vi "writeStatesSamples.vi"(0 "Game in":refnum<class "Game.lvclass">, 1 "Start Recording":bool, 2 "Clear":bool, 3 "Dump":bool, 5 "error in (no error)":errorcluster, 6 "RobotModelFolder":string, 8 "uk":dbl[](array[numeric])) -> (14 "Game out":refnum<class "Game.lvclass">, 19 "error out":errorcluster)   [LabVIEW 2020, in "Game.lvclass"]
uses:
  Game.lvclass
  Game.lvclass/Game.ctl
  Team_class/Team.lvclass/Team.ctl
  Object_class/Object.lvclass/Object.ctl
  Robot_class/Robot.lvclass/Robot.ctl
  Read AllyRef.vi
  Team_class/Read RobotRef.vi
  Object_class/Read x.vi
  Object_class/Read y.vi
  Robot_class/Read orientation.vi
  Ally_class/Ally.lvclass
  C:/Users/anton/Desktop/RoboIME/IC/SSL_AI/Team_class/Team.lvclass
  Robot_class/Robot.lvclass
  C:/Users/anton/Desktop/RoboIME/IC/SSL_AI/Object_class/Object.lvclass
  Utilities_class/Utilities.lvclass
panel:
  out "output array":dbl[][](array[numeric])
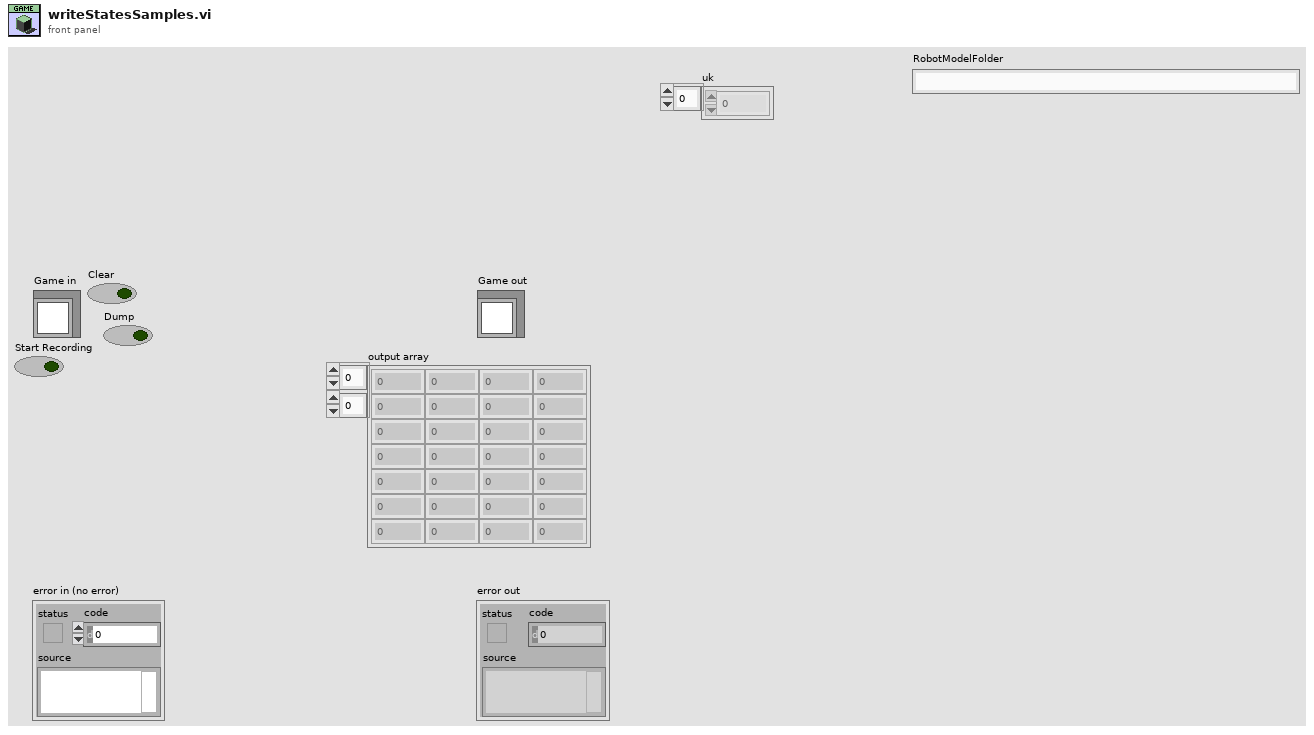
[diagram p1: front panel]
types:
  T1 = cluster{"signal":dbl, "signal":dbl, "signal":dbl}
  T2 = cluster{"signal":dbl, "signal":dbl, "signal":dbl}[]
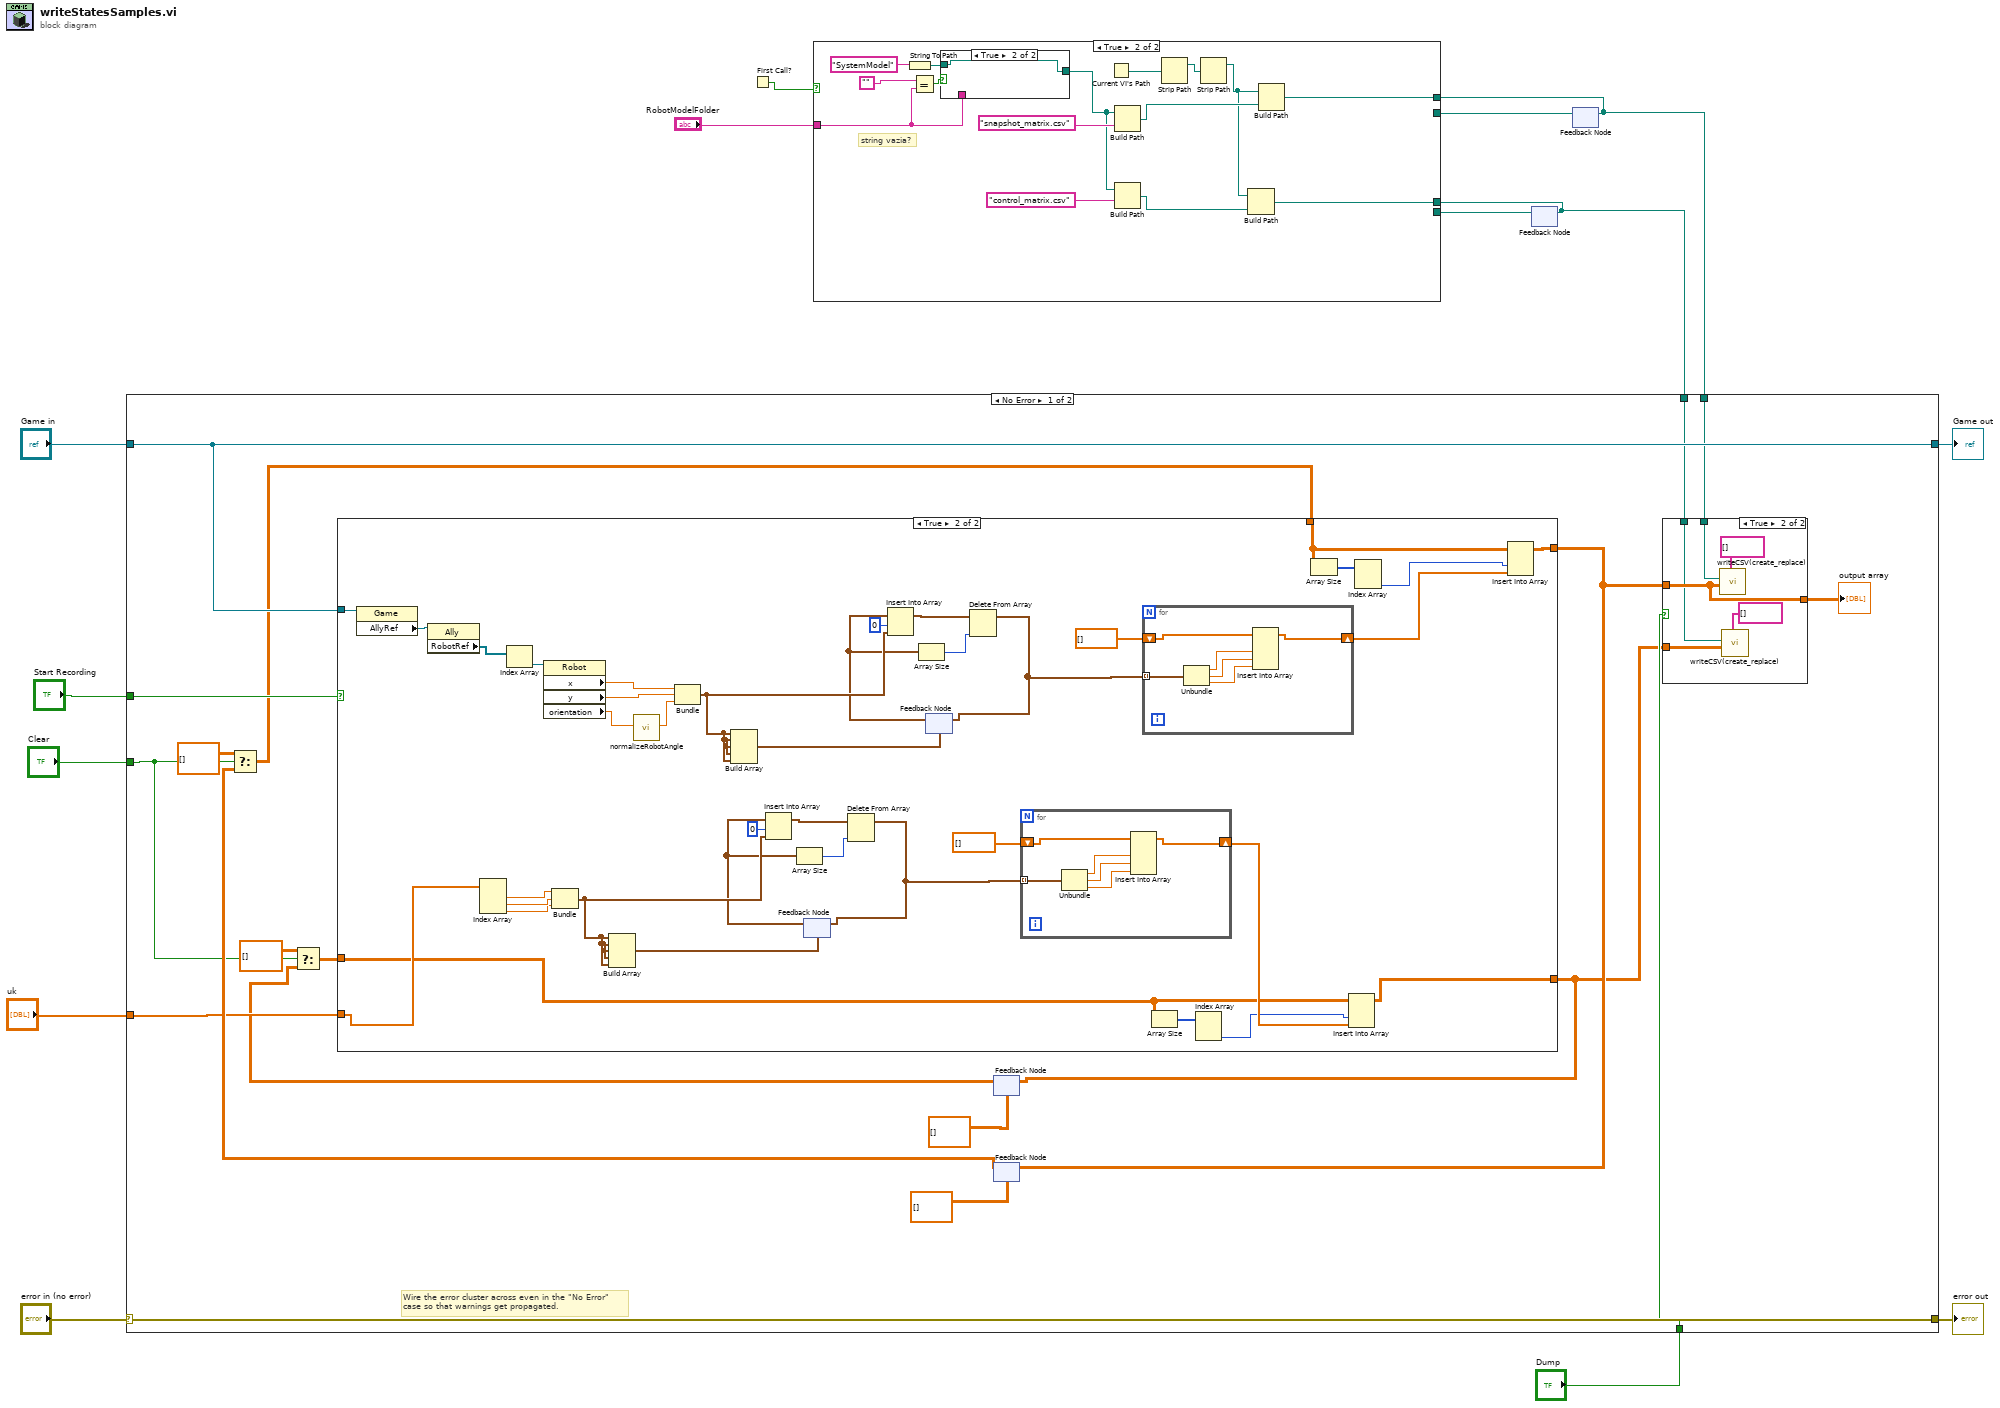
[diagram p0: block diagram]
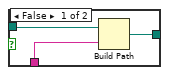
[diagram p3: hidden frame]
diagram:
  n1 = First Call?() -> (First Call?: T/F=w8:bool)
  n2 = feedback #1() -> (w2:path)  [unwired: 1 in]
  n3 = feedback #2() -> (w6:path)  [unwired: 1 in]
  n4 = case shown="True" w8 {
    tunnel: [w16 w29] -> w4
    tunnel: "RobotModelFolder" -> [_ w22]
    tunnel: w6 -> [w16 _]
    tunnel: [w15 w17] -> w1
    tunnel: w2 -> [w15 _]
    frame False {
      # "só precisa calcular o path na 1° iteração"
    }
    frame True {
      # "string vazia?"
      n5 = String To Path(string="SystemModel" ("name or relative path")) -> (path=w23:path)
      n6 = Equal?(x="", y=w22) -> (x = y?=w26:bool)
      n7 = case shown="True" w26 {
        tunnel: w22 -> [w34 _]
        tunnel: [w33 w35] -> w21
        tunnel: w23 -> [w32 w35]
        frame False {
          n8 = Build Path(base path=w32, name or relative path=w34) -> (appended path=w33:path)
        }
        frame True {
        }
      }
      n9 = Current VI's Path() -> (path=w31:path)
      n10 = Build Path(base path=w21, name or relative path="snapshot_matrix.csv") -> (appended path=w27:path)
      n11 = Build Path(base path=w21, name or relative path="control_matrix.csv") -> (appended path=w19:path)
      n12 = Strip Path(path=w31) -> (stripped path=w30:path)  [unwired: 1 out]
      n13 = Strip Path(path=w30) -> (stripped path=w18:path)  [unwired: 1 out]
      n14 = Build Path(base path=w18, name or relative path=w19) -> (appended path=w17:path)
      n15 = Build Path(base path=w18, name or relative path=w27) -> (appended path=w29:path)
    }
  }
  n16 = case shown="No Error" "error in (no error)" {
    selector: "error in (no error)" -> [w54 w115]
    tunnel: [w54 w115] -> w13
    tunnel: [w53 w114] -> w11
    tunnel: "Game in" -> [w53 w114]
    tunnel: "Start Recording" -> [w51 _]
    tunnel: "Clear" -> [w41 _]
    tunnel: "Dump" -> [w48 _]
    tunnel: w4 -> [w47 _]
    tunnel: "uk" -> [w43 _]
    tunnel: w1 -> [w37 _]
    frame No Error {
      # "Wire the error cluster across even in the \"No Error\"\ncase so that warnings get propagated."
      n17 = feedback #3(dbl[][] [] ("appended array")) -> (w40:dbl[][])
      n18 = Select(t=dbl[][] [], s=w41, f=w40) -> (s? t:f=w38:dbl[][])
      n19 = feedback #4(dbl[][] [] ("appended array")) -> (w44:dbl[][])
      n20 = Select(t=dbl[][] [], s=w41, f=w44) -> (s? t:f=w49:dbl[][])
      n21 = case shown="True" w51 {
        tunnel: w53 -> [_ w101]
        tunnel: [w63 w87] -> w46
        tunnel: w49 -> [w63 w86]
        tunnel: w43 -> [_ w69]
        tunnel: w38 -> [w62 w65]
        tunnel: [w62 w64] -> w36
        frame False {
        }
        frame True {
          n22 = property class="Game"(reference=w101) -> ("AllyRef"=w100:refnum<class "Ally.lvclass">)  [unwired: 1 in, 2 out]
          n23 = property class="Ally"(reference=w100) -> ("RobotRef"=w99:refnum<class "Robot.lvclass">[])  [unwired: 1 in, 2 out]
          n24 = Index Array(array=w69) -> (element #1=w68:dbl, element #2=w67:dbl, element #3=w66:dbl)  [unwired: 3 in]
          n25 = Index Array(array=w99) -> (element=w98:refnum<class "Robot.lvclass">)  [unwired: 1 in]
          n26 = property class="Robot"(reference=w98) -> ("x"=w83:dbl, "y"=w97:dbl, "orientation"=w82:dbl)  [unwired: 1 in, 2 out]
          n27 = Bundle("signal"=w68, "signal"=w67, "signal"=w66) -> (w79:T1)  [unwired: 1 in]
          n28 = Build Array(w79, w79, w79, w79, w79) -> (w77:T2)
          n29 = call "normalizeRobotAngle.vi"("signal"=w82) -> ("signal 2"=w81:dbl)  [unwired: 8 in, 2 out]
          n30 = Bundle("x"=w83, "y"=w97, "signal 2"=w81) -> (w95:cluster{"x":dbl, "y":dbl, "signal 2":dbl})  [unwired: 1 in]
          n31 = Build Array(w95, w95, w95, w95, w95) -> (w93:cluster{"x":dbl, "y":dbl, "signal 2":dbl}[])
          n32 = feedback #5(w77) -> (w76:T2)
          n33 = Insert Into Array(array=w76, index=0, new element=w79) -> (w78:T2)
          n34 = Array Size(array=w76) -> (size(s)=w75:i32)
          n35 = Delete From Array(array=w78, index=w75) -> (array with subset deleted=w74:T2)  [unwired: 1 in, 1 out]
          n36 = feedback-in #5(w74) -> ()
          n37 = feedback #6(w93) -> (w92:cluster{"x":dbl, "y":dbl, "signal 2":dbl}[])
          n38 = Insert Into Array(array=w92, index=0, new element=w95) -> (w94:cluster{"x":dbl, "y":dbl, "signal 2":dbl}[])
          n39 = Array Size(array=w92) -> (size(s)=w91:i32)
          n40 = Delete From Array(array=w94, index=w91) -> (array with subset deleted=w90:cluster{"x":dbl, "y":dbl, "signal 2":dbl}[])  [unwired: 1 in, 1 out]
          n41 = feedback-in #6(w90) -> ()
          n42 = for {
            tunnel: w74 -> [w107] mode=indexing
            shift-right: [w105] -> w72
            shift-left: dbl[] [] ("appended array") -> [w106]
            n43 = Unbundle(w107) -> ("signal"=w104:dbl, "signal"=w103:dbl, "signal"=w102:dbl)
            n44 = Insert Into Array(array=w106, new element #1=w104, new element #2=w103, new element #3=w102) -> (w105:dbl[])  [unwired: 1 in]
          }
          n45 = for {
            tunnel: w90 -> [w113] mode=indexing
            shift-right: [w111] -> w88
            shift-left: dbl[] [] ("appended array") -> [w112]
            n46 = Unbundle(w113) -> ("x"=w110:dbl, "y"=w109:dbl, "signal 2"=w108:dbl)
            n47 = Insert Into Array(array=w112, new element #1=w110, new element #2=w109, new element #3=w108) -> (w111:dbl[])  [unwired: 1 in]
          }
          n48 = Array Size(array=w65) -> (size(s)=w71:i32[])
          n49 = Index Array(array=w71) -> (element #2=w70:i32)  [unwired: 2 in, 1 out]
          n50 = Array Size(array=w86) -> (size(s)=w85:i32[])
          n51 = Insert Into Array(array=w65, index (col)=w70, new element=w72) -> (w64:dbl[][])  [unwired: 1 in]
          n52 = Index Array(array=w85) -> (element #2=w84:i32)  [unwired: 2 in, 1 out]
          n53 = Insert Into Array(array=w86, index (col)=w84, new element=w88) -> (w87:dbl[][])  [unwired: 1 in]
        }
      }
      n54 = feedback-in #3(w36) -> ()
      n55 = feedback-in #4(w46) -> ()
      n56 = case shown="True" w48 {
        tunnel: w47 -> [_ w61]
        tunnel: w46 -> [w55 w60]
        tunnel: [w55 w60] -> w45
        tunnel: w37 -> [_ w57]
        tunnel: w36 -> [_ w56]
        frame False {
        }
        frame True {
          n57 = call "writeCSV(create_replace).vi"("Header"=string[] [], "Array"=w60, "file path (use dialog)"=w61) -> ()  [unwired: 7 in, 2 out]
          n58 = call "writeCSV(create_replace).vi"("Header"=string[] [], "Array"=w56, "file path (use dialog)"=w57) -> ()  [unwired: 7 in, 2 out]
        }
      }
      "output array" <- w45
    }
    frame Error {
    }
  }
  "error out" <- w13
  "Game out" <- w11
  n59 = feedback-in #1(w1) -> ()
  n60 = feedback-in #2(w4) -> ()
